vi "finishACBPassPlay.vi"(10 "Game in":refnum<class "Game.lvclass">, 11 "ACBPassPlay in":refnum<class "ACBPassPlay.lvclass">) -> (2 "finishACBPass":bool, 3 "ACBPassPlay out":refnum<class "ACBPassPlay.lvclass">)   [LabVIEW 2020, in "ACBPassPlay.lvclass"]
uses:
  ACBPassPlay.lvclass
  Game_class/Game.lvclass
  C:/Users/anton/Desktop/RoboIME/IC/SSL_AI/Play_class/Play.lvclass
  Referee_class/command_interpreted.ctl
  Game_class/Game.lvclass/Game.ctl
  Events_class/Events.lvclass/Events.ctl
  Ball_class/Ball.lvclass/Ball.ctl
  Referee_class/Referee.lvclass/Referee.ctl
  Team_class/Team.lvclass/Team.ctl
  Game_class/Read Referee.vi
  Referee_class/Read command_interpreted.vi
  Game_class/Read EventsRef.vi
  Game_class/Read BallRef.vi
  Game_class/Read OffensiveTeam.vi
  Team_class/Read RobotRef.vi
  Ball_class/Read z.vi
  Events_class/Read touch.vi
  Events_class/Read id_touch.vi
  Events_class/Read ball_out.vi
  Ally_class/Ally.lvclass
  C:/Users/anton/Desktop/RoboIME/IC/SSL_AI/Team_class/Team.lvclass
  Events_class/Events.lvclass
  Ball_class/Ball.lvclass
  Robot_class/Robot.lvclass
  Referee_class/Referee.lvclass
  Play_class/Play.lvclass
panel:
  out "error out":errorcluster
  in  "error in (no error)":errorcluster
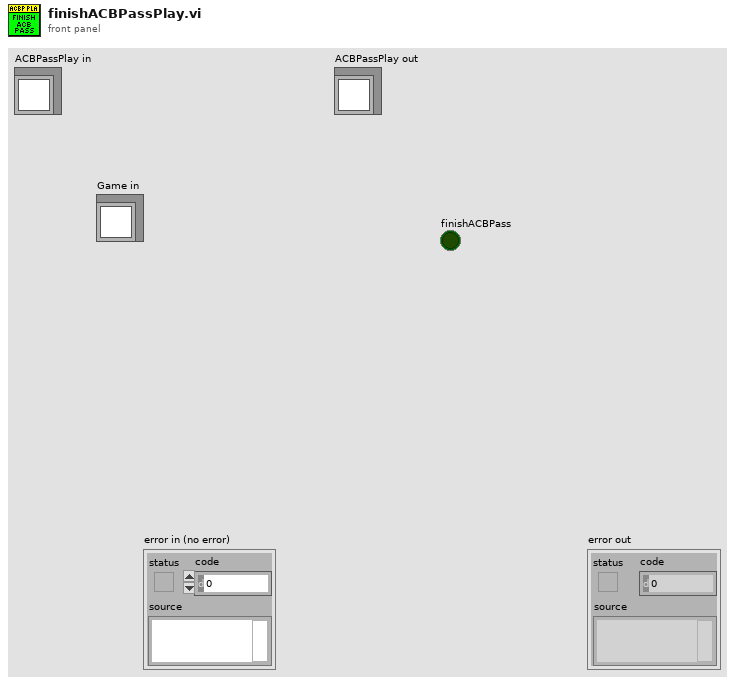
[diagram p1: front panel]
types:
  T1 = typedef "command_interpreted.ctl" = enum16{"Goal Ally", "Goal Enemy", "Ball Placement Enemy", "Ball Placement Ally", "Normal Half Time", "Extra Time  Break", "Extra Half Time", "None", "Post Game", "PKA Normal Start", "Prepare Kickoff Ally", "PKE Normal Start", "Prepare Kickoff Enemy", "Force Start", "Halt", "Timeout", "Prepare Penalty Ally", "Prepare Penalty Enemy", "PPA NormalStart", "PPE Normal Start", "Indirect Free Ally", "Direct Free Enemy", "Direct Free Ally", "Indirect Free Enemy", "Stop"}
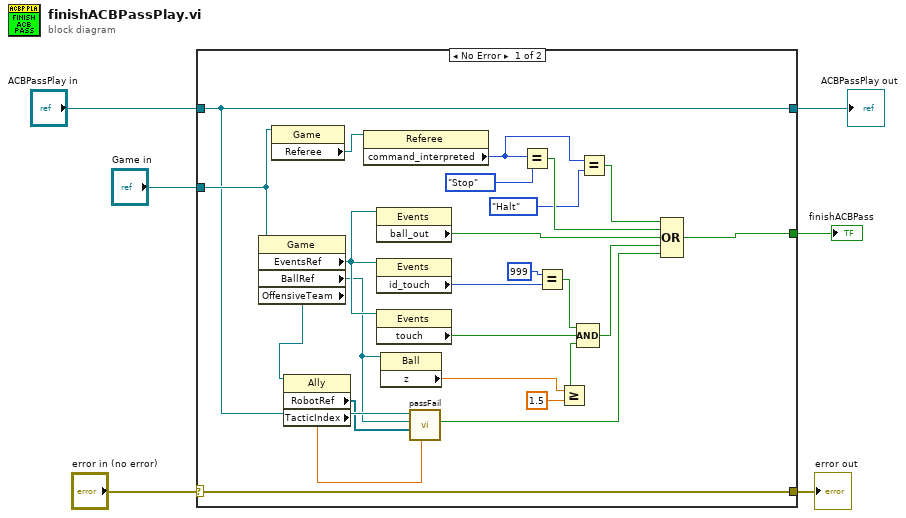
[diagram p0: block diagram]
diagram:
  n1 = case shown="No Error" "error in (no error)" {
    selector: "error in (no error)" -> [w31 w33]
    tunnel: [w31 w33] -> w5
    tunnel: [w15 w32] -> w1
    tunnel: "ACBPassPlay in" -> [w15 w32]
    tunnel: "Game in" -> [w17 _]
    tunnel: [w16 _] -> w3
    frame No Error {
      n2 = property class="Game"(reference=w17) -> ("EventsRef"=w30:refnum<class "Events.lvclass">, "BallRef"=w10:refnum<class "Ball.lvclass">, "OffensiveTeam"=w14:refnum<class "Ally.lvclass">)  [unwired: 1 in, 2 out]
      n3 = property class="Game"(reference=w17) -> ("Referee"=w24:refnum<class "Referee.lvclass">)  [unwired: 1 in, 2 out]
      n4 = property class="Ally"(reference=w14) -> ("RobotRef"=w13:refnum<class "Robot.lvclass">[], "TacticIndex"=w11:dbl)  [unwired: 1 in, 2 out]
      n5 = property class="Referee"(reference=w24) -> ("command_interpreted"=w20:T1)  [unwired: 1 in, 2 out]
      n6 = property class="Events"(reference=w30) -> ("ball_out"=w27:bool)  [unwired: 1 in, 2 out]
      n7 = property class="Events"(reference=w30) -> ("id_touch"=w28:i32)  [unwired: 1 in, 2 out]
      n8 = property class="Events"(reference=w30) -> ("touch"=w23:bool)  [unwired: 1 in, 2 out]
      n9 = property class="Ball"(reference=w10) -> ("z"=w7:dbl)  [unwired: 1 in, 2 out]
      n10 = call "passFail.vi"("TacticIndex"=w11, "Offensive Robots"=w13, "Ball"=w10, "Play in"=w15) -> ("PassFail?"=w12:bool)  [unwired: 5 in, 2 out]
      n11 = Equal?(x=w20, y=command_interpreted."Stop") -> (x = y?=w21:bool)
      n12 = Equal?(x=999 ("id_touch"), y=w28) -> (x = y?=w26:bool)
      n13 = Greater Or Equal?(x=w7, y=1.5) -> (x >= y?=w8:bool)
      n14 = Compound Arithmetic op=AND(w26, w23, w8) -> (w25:bool)
      n15 = Equal?(x=w20, y=command_interpreted."Halt") -> (x = y?=w18:bool)
      n16 = Compound Arithmetic op=OR(w18, w21, w27, w25, w12) -> (w16:bool)
    }
    frame Error {
    }
  }
  "error out" <- w5
  "finishACBPass" <- w3
  "ACBPassPlay out" <- w1
